vi "FootStep_Demo.vi"() -> ()   [LabVIEW 2016]
uses:
  Actuator/Controls/Command cluster.ctl
  Actuator/Controls/Command list.ctl
  General/Controls/data modes.ctl
panel:
  out "Position":dbl(graph)
  in  "Abort":bool
  in  "VISA resource name":refnum<visa-resource-name>="COM4"
  out "Device Information":string
  out "Testing?":bool
  in  "Test":bool
  in  "Speed (mm/s)":dbl=3.0 min=0.1 max=25.0 step=0.1
  out "Position (mm)":dbl
  out "x-y":u32
  out "error out":errorcluster={"status"=FALSE, "code"=1073676294, "source"="VISA Read in SMAC Parameters.vi->SMAC LabVIEW Toolkit_v1.vi"}
  in  "Set point":dbl
  in  "stop":bool
  in  "error in (no error)":errorcluster
  # "Use 'W' and 'S' keys to move the actuator up and down"
  # "- Filename and folder save (metadata + user field)\n- Calibration for load cell"
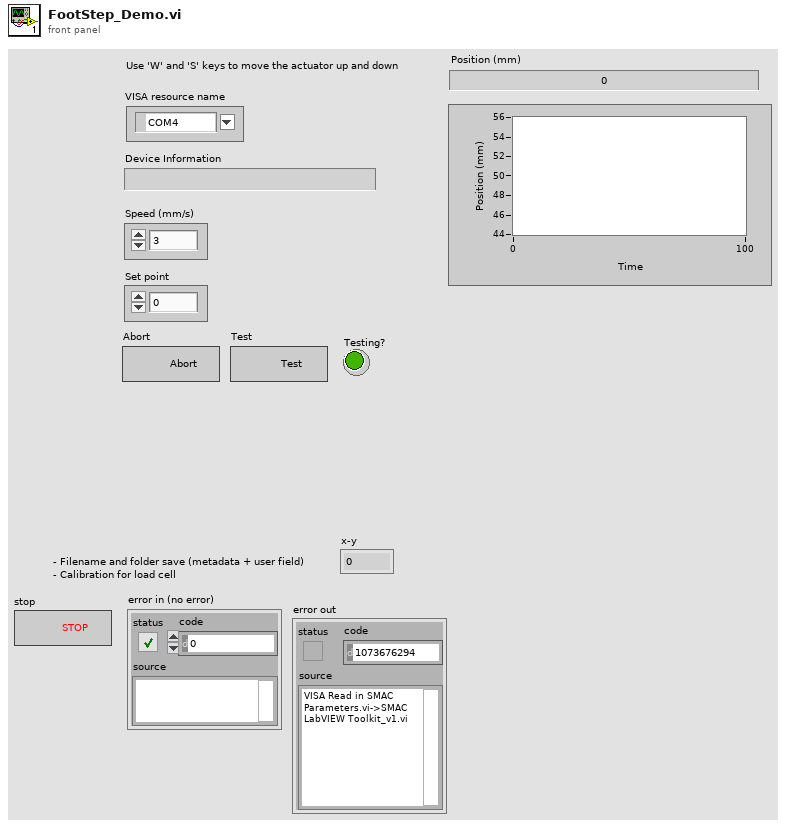
[diagram p1: front panel]
types:
  T1 = typedef "data modes.ctl" = enum16{"Initalise", "Status", "Process", "Add load", "Add position"}
  T2 = typedef "Command cluster.ctl" = cluster{"Command":T3, "data":variant}
  T3 = typedef "Command list.ctl" = enum16{"", "£nabort", "getaxisno", "£getserialno", "£nidentify", "&&£setnlimit", "&£nm", "&£snv", "&£speed", "£np", "£ncal"}
  T4 = cluster{"seconds since 1Jan1904":timestamp, "data":dbl}[]
  T5 = cluster{"seconds since 1Jan1904":timestamp, "data":dbl}
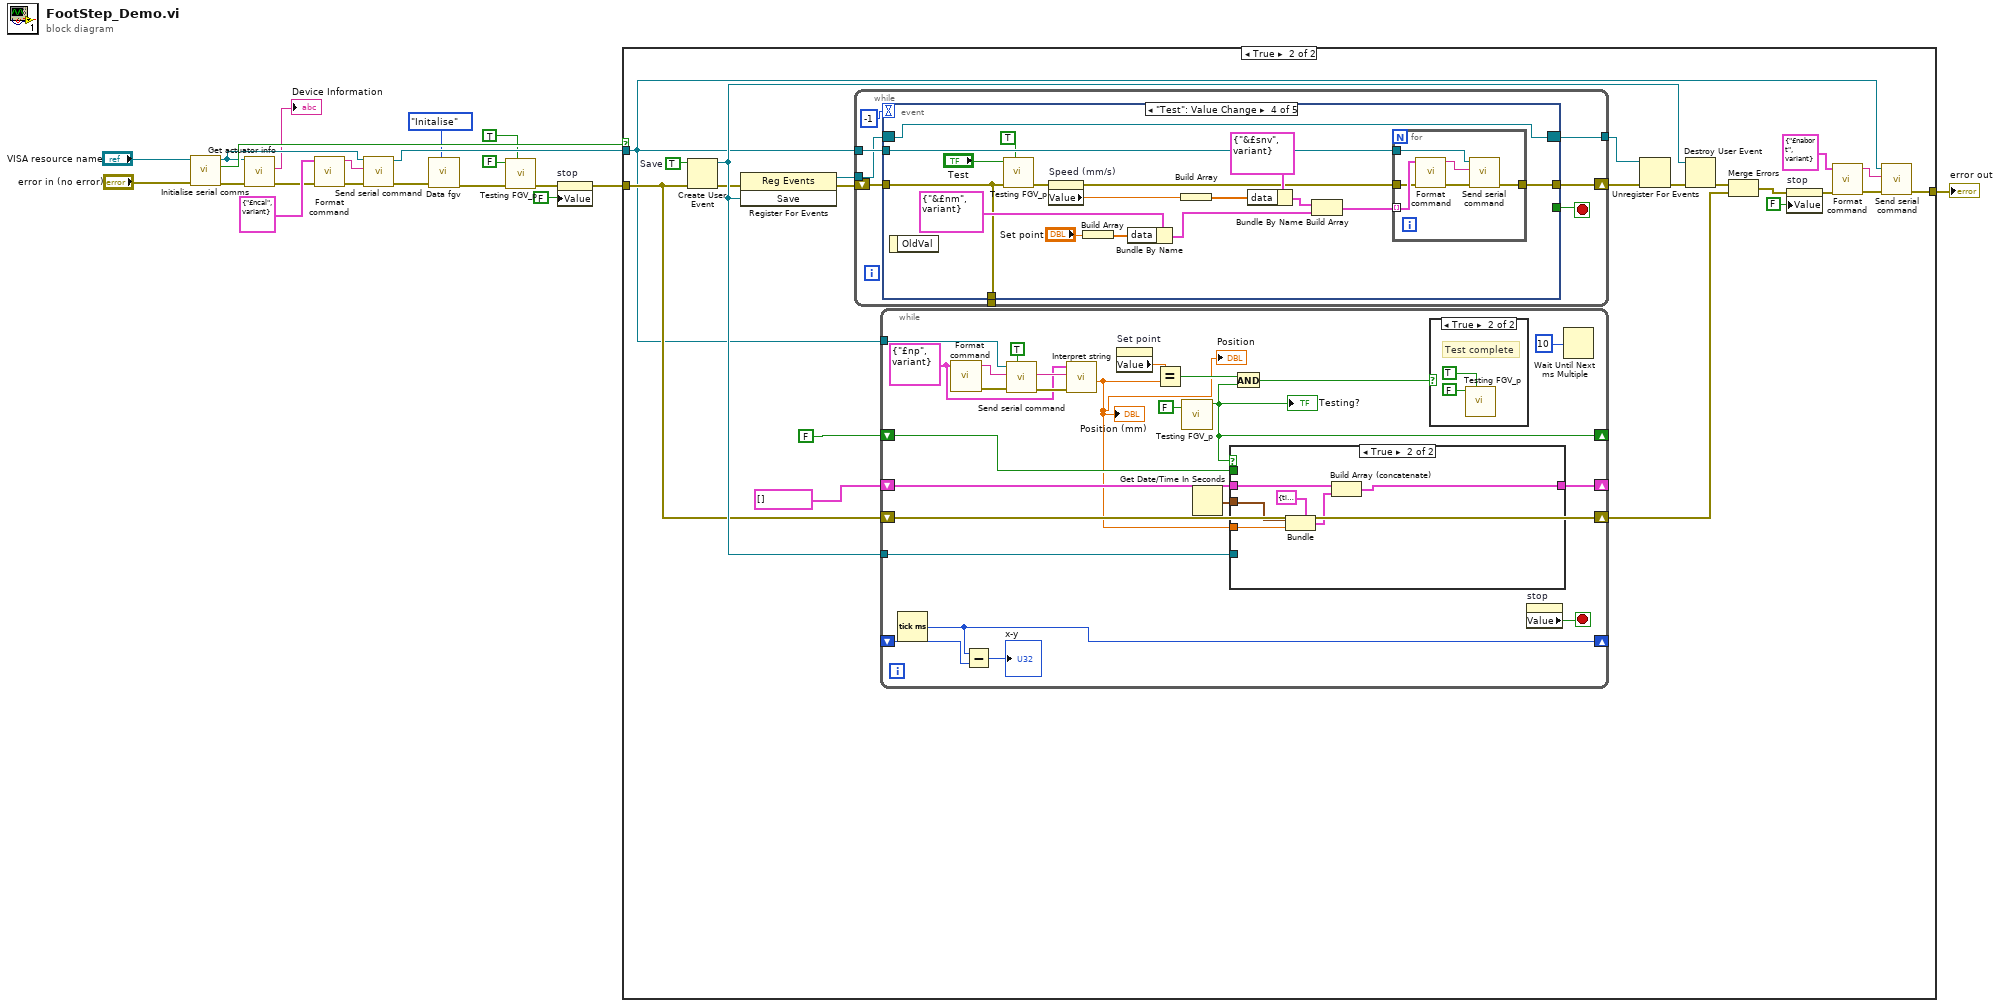
[diagram p0: block diagram]
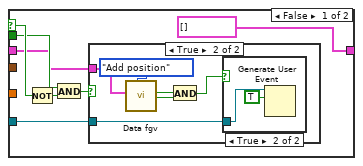
[diagram p3: hidden frame]
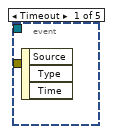
[diagram p7: hidden frame]
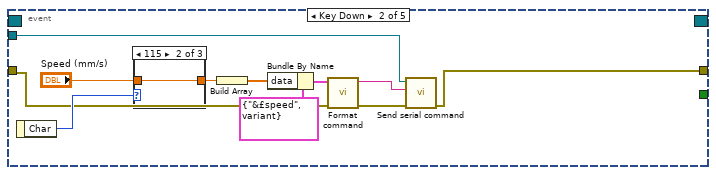
[diagram p8: hidden frame]
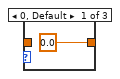
[diagram p9: hidden frame]
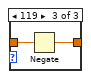
[diagram p10: hidden frame]
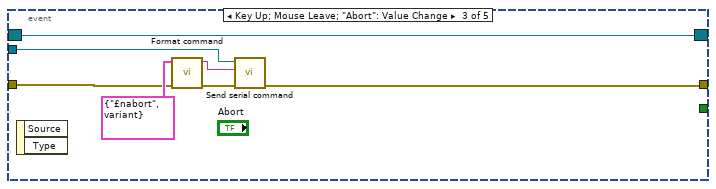
[diagram p11: hidden frame]
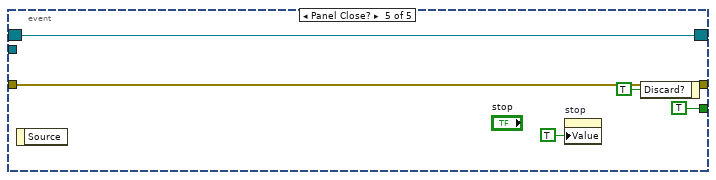
[diagram p12: hidden frame]
diagram:
  n1 = call "Initialise serial comms.vi"("error in (no error)"="error in (no error)", "VISA Refnum in"="VISA resource name") -> ("error out"=w20:errorcluster, "Connected?"=w14:bool, "VISA Refnum out"=w13:refnum<visa-resource-name>)  [unwired: 7 in]
  n2 = call "Get actuator info.vi"("error in (no error)"=w20, "VISA Refnum in"=w13) -> ("error out"=w17:errorcluster, "String"=→"Device Information":string)  [unwired: 7 in, 1 out]
  n3 = call "Format command.vi"("error in (no error)"=w17, "Cluster"=T2 {"Command"=enum."£ncal", "data"=variant}) -> ("error out"=w16:errorcluster, "String"=w15:string)  [unwired: 8 in]
  n4 = call "Send serial command.vi"("error IO"=w16, "Send string"=w15, "VISA resource name out"=w13) -> ("error out"=w8:errorcluster, "VISA Out"=w12:refnum<visa-resource-name>)  [unwired: 6 in, 1 out]
  n5 = call "Data fgv.vi"("Modes"=data_modes."Initalise", "error in (no error)"=w8) -> ("error out"=w7:errorcluster)  [unwired: 5 in, 4 out]
  n6 = call "Testing FGV_p.vi"("Set"=TRUE, "error in (no error)"=w7, "Value"=FALSE) -> ("error out"=w6:errorcluster)  [unwired: 7 in, 1 out]
  n7 = property on="stop" class="Bool (strict)"(error in=w6, "Value"=FALSE ("stop")) -> (error out=w5:errorcluster)  [unwired: 1 in, 1 out]
  n8 = case shown="True" w14 {
    tunnel: w12 -> [_ w22]
    tunnel: w5 -> [w21 w28]
    tunnel: [w21 w23] -> w3
    frame False {
    }
    frame True {
      w40 = TRUE  # Save
      n9 = Create User Event(user event datatype=w40, error in=w28) -> (user event=w36:refnum<user-event>, error out=w35:errorcluster)
      n10 = register-events(error in=w35, w36) -> (reference out=w39:refnum<event-registration>, error out=w34:errorcluster)  [unwired: 1 in]
      n11 = while {
        tunnel: w22 -> [w96]
        tunnel: [w94] -> _
        tunnel: w39 -> [w93]
        tunnel: [w92] -> w38
        shift-right: [w90] -> w33
        shift-left: w34 -> [w95]
        stop <- w91 stop-if-true
        n12 = event shown="[3] \"Test\": Value Change" {
          selector: w93 -> [_ _ w113 w120 w146]
          dyn-events: [_ _ w113 w120 w146] -> w92
          timeout: -1 -> [_ _ _ _ _]
          tunnel: w96 -> [_ w103 w117 w135 _]
          tunnel: w95 -> [_ w99 w115 w124 w145]
          tunnel: [_ _ _ w124 _] -> w94
          tunnel: [_ _ _ _ TRUE] -> w91
          tunnel: [_ w98 w114 w121 w145] -> w90
          event Timeout {
            n13 = event-data() -> ()  [unwired: 1 in, 3 out]
          }
          event Key Down {
            n14 = event-data() -> ("Char"=w102:i16)  [unwired: 1 in]
            n15 = case shown="115" w102 {
              tunnel: [0.0 w110 w112] -> w107
              tunnel: "Speed (mm/s)" -> [_ w110 w111]
              frame 0, Default {
              }
              frame 115 {
              }
              frame 119 {
                n16 = Negate(x=w111) -> (-x=w112:dbl)
              }
            }
            n17 = Build Array(w107) -> (w106:dbl[])
            n18 = Bundle By Name(cluster=T2 {"Command"=enum."&£speed", "data"=variant} ("Cluster"), "data"=w106) -> (w105:T2)
            n19 = call "Format command.vi"("error in (no error)"=w99, "Cluster"=w105) -> ("error out"=w100:errorcluster, "String"=w104:string)  [unwired: 8 in]
            n20 = call "Send serial command.vi"("error IO"=w100, "Send string"=w104, "VISA resource name out"=w103) -> ("error out"=w98:errorcluster)  [unwired: 6 in, 2 out]
          }
          event Key Up; Mouse Leave; "Abort": Value Change {
            n21 = event-data() -> ()  [unwired: 1 in, 2 out]
            n22 = call "Format command.vi"("error in (no error)"=w115, "Cluster"=T2 {"Command"=enum."£nabort", "data"=variant} ("Cluster 2")) -> ("error out"=w118:errorcluster, "String"=w119:string)  [unwired: 8 in]
            n23 = call "Send serial command.vi"("error IO"=w118, "Send string"=w119, "VISA resource name out"=w117) -> ("error out"=w114:errorcluster)  [unwired: 6 in, 2 out]
          }
          event "Test": Value Change {
            n24 = event-data() -> ()  [unwired: 1 in, 1 out]
            n25 = call "Testing FGV_p.vi"("Set"=TRUE, "error in (no error)"=w124, "Value"="Test") -> ("error out"=w123:errorcluster)  [unwired: 7 in, 1 out]
            n26 = property on="Speed (mm/s)" class="DigNum (strict)"(error in=w123) -> (error out=w122:errorcluster, "Value"=w127:dbl)  [unwired: 1 in, 1 out]
            n27 = Build Array("Set point") -> (w130:dbl[])
            n28 = Bundle By Name(cluster=T2 {"Command"=enum."&£nm", "data"=variant} ("Cluster"), "data"=w130) -> (w129:T2)
            n29 = Build Array(w127) -> (w128:dbl[])
            n30 = Bundle By Name(cluster=T2 {"Command"=enum."&£snv", "data"=variant} ("Cluster"), "data"=w128) -> (w132:T2)
            n31 = Build Array(w132, w129) -> (w134:T2[])
            n32 = for {
              tunnel: w135 -> [w141]
              tunnel: w134 -> [w139] mode=indexing
              tunnel: w122 -> [w138]
              tunnel: [w137] -> w121
              n33 = call "Format command.vi"("error in (no error)"=w138, "Cluster"=w139) -> ("error out"=w142:errorcluster, "String"=w140:string)  [unwired: 8 in]
              n34 = call "Send serial command.vi"("error IO"=w142, "Send string"=w140, "VISA resource name out"=w141) -> ("error out"=w137:errorcluster)  [unwired: 6 in, 2 out]
            }
          }
          event Panel Close? {
            n35 = event-data() -> ()  [unwired: 1 in, 1 out]
            n36 = property on="stop" class="Bool (strict)"("Value"=TRUE ("stop")) -> ()  [unwired: 2 in, 2 out]
            n37 = event-data("Discard?"=TRUE) -> ()  [unwired: 1 in, 1 out]
          }
        }
      }
      n38 = while {
        tunnel: w22 -> [w64]
        shift-right: [w62] -> _
        shift-left: _ -> [w61]
        shift-right: [w50] -> _
        shift-left: T4 [] ("Data") -> [w54]
        shift-right: [w51] -> _
        shift-left: FALSE ("Testing?") -> [w52]
        tunnel: w36 -> [w49]
        shift-right: [w48] -> w29
        shift-left: w28 -> [w48]
        stop <- w47 stop-if-true
        w44 = T2 {"Command"=enum."£np", "data"=variant} ("Cluster")
        n39 = Tick Count (ms)() -> (millisecond timer value=w62:u32)
        n40 = call "Format command.vi"("Cluster"=w44) -> ("error out"=w46:errorcluster, "String"=w65:string)  [unwired: 9 in]
        n41 = Subtract(x=w62, y=w61) -> (x-y=→"x-y":u32)
        n42 = call "Send serial command.vi"("Read?"=TRUE, "error IO"=w46, "Send string"=w65, "VISA resource name out"=w64) -> ("error out"=w45:errorcluster, "read string"=w59:string)  [unwired: 5 in, 1 out]
        n43 = call "Interpret string.vi"("error in (no error)"=w45, "String"=w59, "Cluster"=w44) -> ("Numeric 2"=w43:dbl)  [unwired: 5 in, 3 out]
        "Position (mm)" <- w43
        "Position" <- w43
        n44 = property on="Set point" class="DigNum (strict)"() -> ("Value"=w58:dbl)  [unwired: 2 in, 2 out]
        n45 = Equal?(x=w58, y=w43) -> (x = y?=w57:bool)
        n46 = call "Testing FGV_p.vi"("Set"=FALSE) -> ("Testing?"=w51:bool)  [unwired: 9 in, 1 out]
        "Testing?" <- w51
        n47 = Get Date/Time In Seconds() -> (seconds since 1Jan1904=w53:timestamp)
        n48 = case shown="True" w51 {
          selector: w51 -> [w72 _]
          tunnel: w53 -> [_ w86]
          tunnel: w43 -> [_ w85]
          tunnel: w52 -> [w70 _]
          tunnel: w54 -> [w69 w84]
          tunnel: [T4 [] w82] -> w50
          tunnel: w49 -> [w67 _]
          frame False {
            n49 = Not(x=w72) -> (.not. x?=w71:bool)
            n50 = And(x=w70, y=w71) -> (x .and. y?=w68:bool)
            n51 = case shown="True" w68 {
              tunnel: w69 -> [_ w78]
              tunnel: w67 -> [_ w74]
              frame False {
              }
              frame True {
                n52 = call "Data fgv.vi"("Modes"=data_modes."Add position", "Data"=w78) -> ("Load?"=w76:bool, "Position?"=w77:bool)  [unwired: 5 in, 3 out]
                n53 = And(x=w77, y=w76) -> (x .and. y?=w75:bool)
                n54 = case shown="True" w75 {
                  tunnel: w74 -> [_ w81]
                  frame False {
                  }
                  frame True {
                    n55 = Generate User Event(user event=w81, event data cluster=TRUE ("event data")) -> ()  [unwired: 2 in, 2 out]
                  }
                }
              }
            }
          }
          frame True {
            n56 = Bundle(cluster=T5 {"seconds since 1Jan1904"=timestamp(0 s since 1904-01-01), "data"=0.0} ("element"), "seconds since 1Jan1904"=w86, "data"=w85) -> (w83:T5)
            n57 = Build Array (concatenate)(w84, w83) -> (w82:T4)
          }
        }
        n58 = And(x=w57, y=w51) -> (x .and. y?=w55:bool)
        n59 = case shown="True" w55 {
          frame False {
          }
          frame True {
            # "Test complete"
            n60 = call "Testing FGV_p.vi"("Set"=TRUE, "Value"=FALSE) -> ()  [unwired: 8 in, 2 out]
          }
        }
        n61 = property on="stop" class="Bool (strict)"() -> ("Value"=w47:bool)  [unwired: 2 in, 2 out]
        n62 = Wait Until Next ms Multiple(millisecond multiple=u32 10) -> ()  [unwired: 1 out]
      }
      n63 = Unregister For Events(event registration refnum=w38, error in=w33) -> (error out=w37:errorcluster)
      n64 = Destroy User Event(user event=w36, error in=w37) -> (error out=w32:errorcluster)
      n65 = Merge Errors(w32, w29) -> (w31:errorcluster)
      n66 = property on="stop" class="Bool (strict)"(error in=w31, "Value"=FALSE ("stop")) -> (error out=w24:errorcluster)  [unwired: 1 in, 1 out]
      n67 = call "Format command.vi"("error in (no error)"=w24, "Cluster"=T2 {"Command"=enum."£nabort", "data"=variant} ("Cluster 2")) -> ("error out"=w25:errorcluster, "String"=w26:string)  [unwired: 8 in]
      n68 = call "Send serial command.vi"("error IO"=w25, "Send string"=w26, "VISA resource name out"=w22) -> ("error out"=w23:errorcluster)  [unwired: 6 in, 2 out]
    }
  }
  "error out" <- w3
